vi "Dialog_SetBlockTo.vi"(4 "ModeCol Index":i32=2, 6 "Cell Position":T1, 7 "Table History ref":refnum<vi>, 8 "error in (no error)":errorcluster, 9 "Table CtlRef In":refnum<vi>, 10 "VariableManagerRef":refnum<vi>, 11 "Col Array Ref in":refnum<vi>) -> (0 "error out":errorcluster, 2 "OK":bool)   [LabVIEW 2013]
doc: "Apply a user selected value to the entire block-selection in the \"Table CtlRef In.\" The user will be prompted to choose between entering a value, adding a variable (pre-populated based on which cell the user actually clicked), or selecting one of the values within the block. If the user makes a change, theTable History is also updated."
uses:
  TypeDefs/TableHistory.ctl
  TypeDefs/TableArray.ctl
  <vilib>/Utility/miscctls.llb/LVRowAndColumnTypeDef.ctl
  VariableManagerCodes/VariableManager/VariableManager.lvclass
  <vilib>/Utility/cursorutil.llb/Set Cursor (Icon Pict).vi
panel:
  out "chosen":string
  out "Unique List":string[](array[string])
  in  "Cancel":bool
  in  "SetTo:":i32(ring) items=["<Select value...>", "Add variable...", "Other value...", "1", "0"]
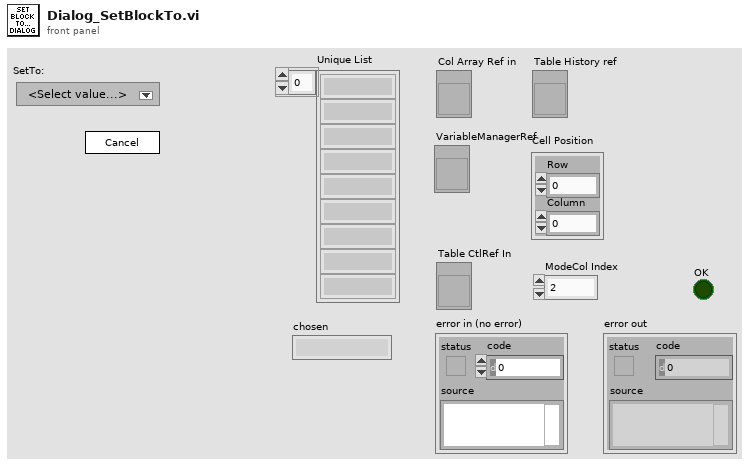
[diagram p1: front panel]
types:
  T1 = typedef "LVRowAndColumnTypeDef.ctl" = cluster{"Row":i32, "Column":i32}
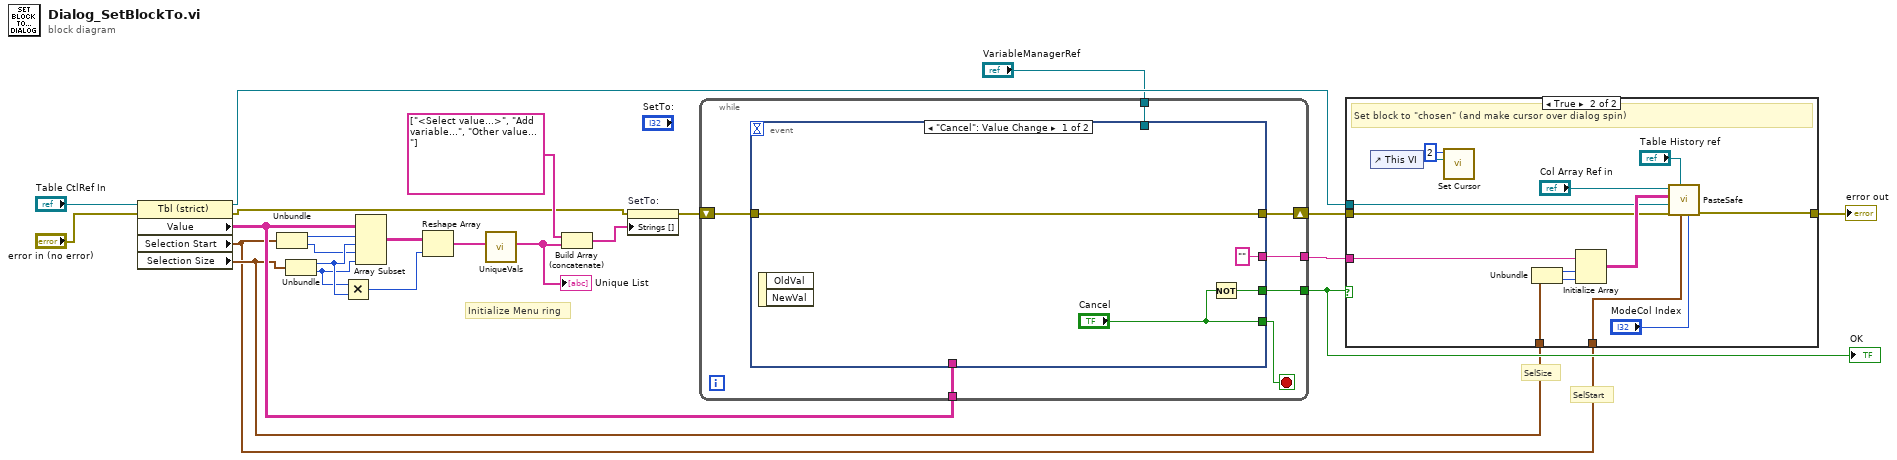
[diagram p0: block diagram]
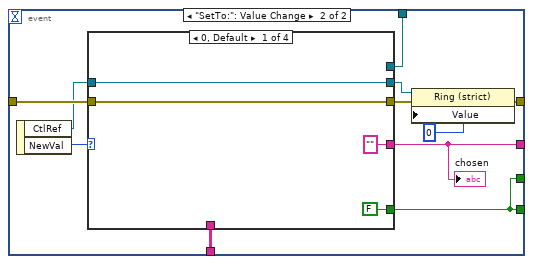
[diagram p3: hidden frame]
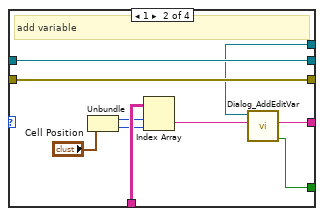
[diagram p4: hidden frame]
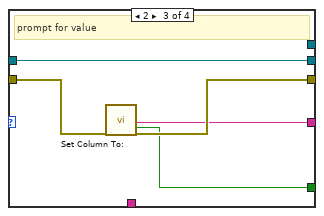
[diagram p5: hidden frame]
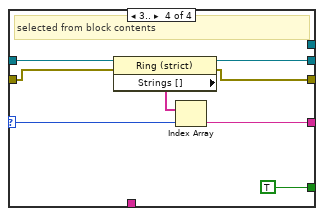
[diagram p6: hidden frame]
diagram:
  # "SelStart"
  # "SelSize"
  # "Initialize Menu ring"
  n1 = property class="Tbl (strict)"(reference="Table CtlRef In", error in="error in (no error)") -> (reference out=w3:refnum<vi>, error out=w2:errorcluster, "Value"=w6:string[][], "Selection Start"=w4:T1, "Selection Size"=w5:T1)
  n2 = Unbundle(w4) -> ("Row"=w21:i32, "Column"=w10:i32)
  n3 = Unbundle(w5) -> ("Row"=w18:i32, "Column"=w9:i32)
  n4 = Multiply(x=w9, y=w18) -> (x*y=w17:i32)
  n5 = Array Subset(array=w6, index (row)=w21, length (row)=w18, index (col)=w10, length (col)=w9) -> (w20:string[][])
  n6 = Reshape Array(w20, w17) -> (w19:string[])
  n7 = call "UniqueVals.vi"("Array in"=w19) -> ("Unique List"=w16:string[])  [unwired: 10 in]
  "Unique List" <- w16
  n8 = Build Array (concatenate)(string[] ["<Select value...>", "Add variable...", "Other value..."] ("element"), w16) -> (w14:string[])
  n9 = property on="SetTo:" class="Ring (strict)"(error in=w2, "Strings []"=w14) -> (error out=w13:errorcluster)  [unwired: 1 in, 1 out]
  n10 = while {
    shift-right: [w28] -> w12
    shift-left: w13 -> [w29]
    tunnel: [w27] -> w7
    tunnel: [w26] -> w8
    tunnel: w6 -> [w25]
    tunnel: "VariableManagerRef" -> [w24]
    stop <- w30 stop-if-true
    n11 = event shown="[0] \"Cancel\": Value Change" {
      selector: _ -> [_ _]
      dyn-events: _ -> [_ _]
      timeout: _ -> [_ _]
      tunnel: ["Cancel" w37] -> w30
      tunnel: w29 -> [w34 w44]
      tunnel: [w34 w41] -> w28
      tunnel: ["" ("value") w38] -> w27
      tunnel: [w31 w37] -> w26
      tunnel: w25 -> [_ w36]
      tunnel: w24 -> [_ w35]
      event "Cancel": Value Change {
        n12 = event-data() -> ()  [unwired: 1 in, 2 out]
        n13 = Not(x="Cancel") -> (.not. x?=w31:bool)
      }
      event "SetTo:": Value Change {
        n14 = event-data() -> ("CtlRef"=w43:refnum<vi>, "NewVal"=w45:i32)  [unwired: 1 in]
        n15 = case shown="0, Default" w45 {
          selector: w45 -> [_ _ _ w69]
          tunnel: w43 -> [w48 w55 w64 w72]
          tunnel: w44 -> [w49 w54 w63 w71]
          tunnel: [w49 w54 w62 w68] -> w42
          tunnel: ["" ("Variable Name") w59 w60 w67] -> w38
          tunnel: [FALSE ("OK?") w58 w61 TRUE ("OK")] -> w37
          tunnel: [w48 w55 w64 w66] -> w40
          tunnel: w36 -> [_ w53 _ _]
          tunnel: w35 -> [_ w50 _ _]
          frame 0, Default {
          }
          frame 1 {
            # "add variable"
            n16 = Unbundle("Cell Position") -> ("Row"=w52:i32, "Column"=w51:i32)
            n17 = Index Array(array=w53, index (row)=w52, index (col)=w51) -> (element=w56:string)
            n18 = call "Dialog_AddEditVar.vi"("String in"=w56, "VariableManagerRef"=w50) -> ("OK?"=w58:bool, "Variable Name"=w59:string)  [unwired: 8 in]
          }
          frame 2 {
            # "prompt for value"
            n19 = call "Set Column To:"("error in (no error)"=w63) -> ("value"=w60:string, "OK"=w61:bool, "error out"=w62:errorcluster)  [unwired: 16 in]
          }
          frame 3.. {
            # "selected from block contents"
            n20 = property class="Ring (strict)"(reference=w72, error in=w71) -> (reference out=w66:refnum<vi>, error out=w68:errorcluster, "Strings []"=w70:string[])
            n21 = Index Array(array=w70, index=w69) -> (element=w67:string)
          }
        }
        "chosen" <- w38
        n22 = property class="Ring (strict)"(reference=w40, error in=w42, "Value"=0) -> (error out=w41:errorcluster)  [unwired: 1 out]
      }
    }
  }
  "OK" <- w8
  n23 = case shown="True" w8 {
    tunnel: w12 -> [w73 w76]
    tunnel: [w73 w77] -> w11
    tunnel: w7 -> [_ w86]
    tunnel: w5 -> [_ w87]
    tunnel: w4 -> [_ w80]
    tunnel: w3 -> [_ w78]
    frame False {
      # "user cancelled."
    }
    frame True {
      # "Set block to \"chosen\" (and make cursor over dialog spin)"
      n24 = control-ref of="This VI"() -> (w75:refnum<vi>)
      n25 = call-poly <vilib>:"Set Cursor.vi"("VI reference (current VI)"=w75, "icon"=u16 2) -> ()  [unwired: 8 in, 2 out]
      n26 = Unbundle(w87) -> ("Row"=w84:i32, "Column"=w85:i32)
      n27 = Initialize Array(w86, w84, w85) -> (w83:string[][])
      n28 = call "PasteSafe.vi"("ModeCol Index"="ModeCol Index", "Cell Start"=w80, "Table History ref"="Table History ref", "error in (no error)"=w76, "Table CtlRef In"=w78, "Clipboard (clipped)"=w83, "Col Array Ref in"="Col Array Ref in") -> ("error out"=w77:errorcluster)  [unwired: 2 in, 2 out]
    }
  }
  "error out" <- w11
